vi "UnInstall.vi"   [LabVIEW 2014]
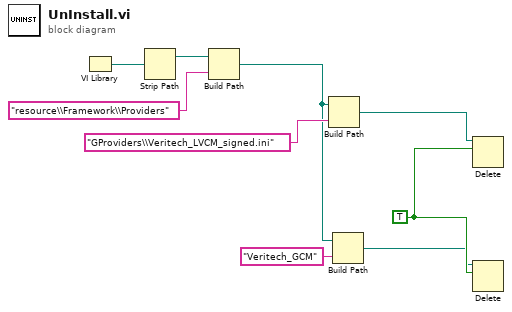
[diagram p0: block diagram]
diagram:
  w4 = TRUE ("overwrite (F)")
  n1 = VI Library() -> (path=w9:path)
  n2 = Strip Path(path=w9) -> (stripped path=w8:path)  [unwired: 1 out]
  n3 = Build Path(base path=w8, name or relative path="resource\\Framework\\Providers") -> (appended path=w2:path)
  n4 = Build Path(base path=w2, name or relative path="GProviders\\Veritech_LVCM_signed.ini") -> (appended path=w5:path)
  n5 = Build Path(base path=w2, name or relative path="Veritech_GCM") -> (appended path=w1:path)
  n6 = Delete(path (use dialog)=w5, entire hierarchy (F)=w4) -> ()  [unwired: 3 in, 3 out]
  n7 = Delete(path (use dialog)=w1, entire hierarchy (F)=w4) -> ()  [unwired: 3 in, 3 out]
